vi "Local UV_Serial Link.vi"(8 "error in":errorcluster, 9 "data bits (8)":u16=8, 10 "baud rate (9600)":u32=9600, 11 "VISA resource name":refnum<visa-resource-name>="COM5") -> (0 "error out":errorcluster, 3 "VISA resource out":refnum<visa-resource-name>)   [LabVIEW 2018]
uses:
  <vilib>/Instr/_visa.llb/VISA Configure Serial Port (Instr).vi
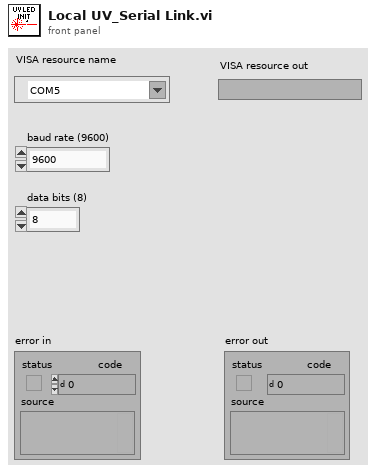
[diagram p1: front panel]
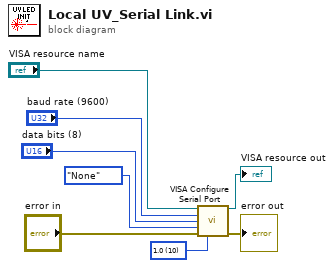
[diagram p0: block diagram]
diagram:
  w5 = u16 10 items=["1.0"=10, "1.5"=15, "2.0"=20] ("stop bits (10: 1 bit)")
  n1 = call-poly "VISA Configure Serial Port"("VISA resource name"="VISA resource name", "baud rate (9600)"="baud rate (9600)", "data bits (8)"="data bits (8)", "parity (0:none)"=enum16{"None", "Odd", "Even", "Mark", "Space"}."None", "error in (no error)"="error in", "stop bits (10: 1 bit)"=w5) -> ("VISA resource name out"=→"VISA resource out":refnum<visa-resource-name>, "error out"=→"error out":errorcluster)  [unwired: 8 in]
